vi "WRITE_xlsx.vi"(7 "是否下一行输入？":bool, 8 "错误输入（无错误）":errorcluster, 9 "输入内容":string[][](array[string]), 10 "输入列字母":string, 11 "该文档引用输入":refnum<k7>) -> (0 "错误输出":errorcluster)   [LabVIEW 2014]
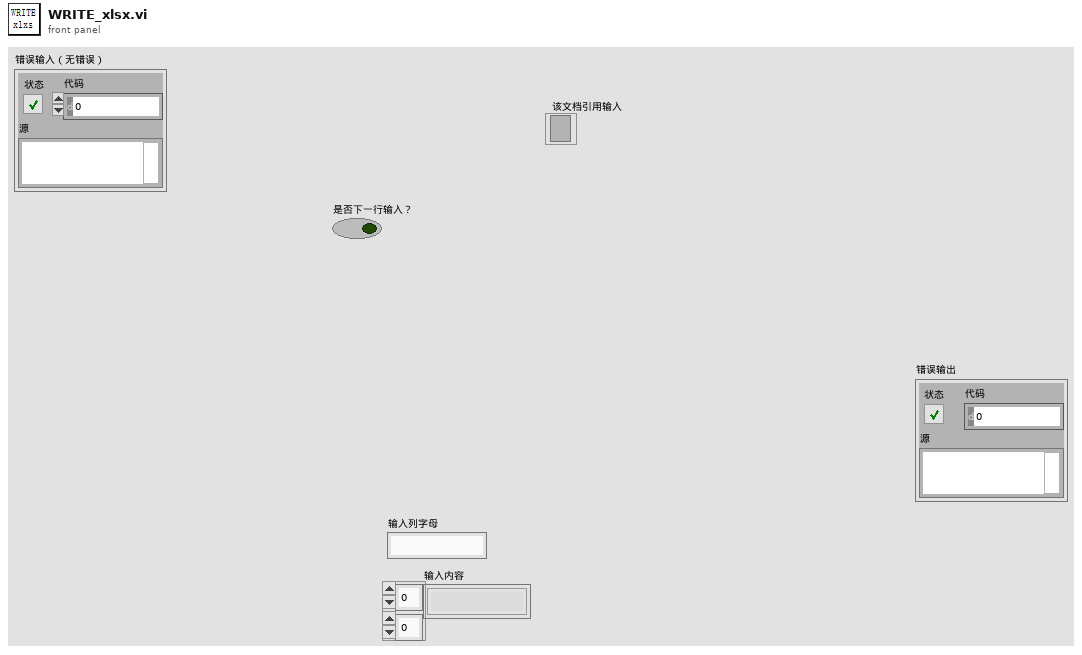
[diagram p1: front panel]
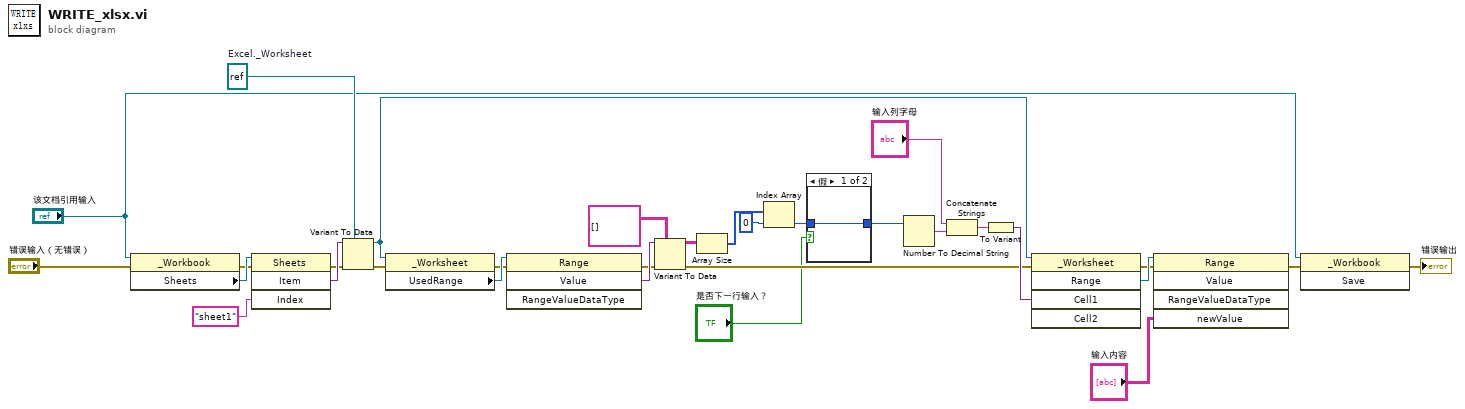
[diagram p0: block diagram]
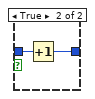
[diagram p2: hidden frame]
diagram:
  w28 = refnum<k7> refnum  # Excel._Worksheet
  n1 = property class="_Workbook"(reference="该文档引用输入", error in="错误输入（无错误）") -> (error out=w26:errorcluster, "Sheets"=w31:refnum<k7>)  [unwired: 1 out]
  n2 = invoke class="Sheets" method="Item"(reference=w31, error in=w26, "Index"="sheet1" ("字符串")) -> (error out=w27:errorcluster, "Item"=w29:variant)  [unwired: 1 in, 2 out]
  n3 = Variant To Data(error in=w27, type=w28, Variant=w29) -> (data=w14:refnum<k7>, error out=w25:errorcluster)
  n4 = property class="_Worksheet"(reference=w14, error in=w25) -> (error out=w23:errorcluster, "UsedRange"=w24:refnum<k7>)  [unwired: 1 out]
  n5 = invoke class="Range" method="Value"(reference=w24, error in=w23) -> (error out=w21:errorcluster, "Value"=w22:variant)  [unwired: 2 in, 2 out]
  n6 = Variant To Data(error in=w21, type=string[][] [] ("数组"), Variant=w22) -> (data=w19:string[][], error out=w11:errorcluster)
  n7 = Array Size(array=w19) -> (size(s)=w18:i32[])
  n8 = Index Array(array=w18, index=0 ("索引")) -> (element=w3:i32)
  n9 = case shown="假" "是否下一行输入？" {
    tunnel: w3 -> [w32 w34]
    tunnel: [w32 w33] -> w2
    frame False {
    }
    frame True {
      n10 = Increment(x=w34) -> (x+1=w33:i32)
    }
  }
  n11 = Number To Decimal String(number=w2) -> (decimal integer string=w8:string)  [unwired: 1 in]
  n12 = Concatenate Strings("输入列字母", w8) -> (w10:string)
  n13 = To Variant(anything=w10) -> (Variant=w13:variant)
  n14 = invoke class="_Worksheet" method="Range"(reference=w14, error in=w11, "Cell1"=w13) -> (error out=w15:errorcluster, "Range"=w16:refnum<k7>)  [unwired: 2 in, 3 out]
  n15 = invoke class="Range" method="Value"(reference=w16, error in=w15, "newValue"="输入内容") -> (error out=w6:errorcluster)  [unwired: 2 in, 4 out]
  n16 = invoke class="_Workbook" method="Save"(reference="该文档引用输入", error in=w6) -> (error out=→"错误输出":errorcluster)  [unwired: 1 in, 2 out]
